vi "read position.vi"(8 "error in (no error)":errorcluster, 11 "Stepper in":refnum<class "Stepper.lvclass">) -> (0 "error out":errorcluster, 2 "Angle":dbl, 3 "Stepper out":refnum<class "Stepper.lvclass">)   [LabVIEW 2025, in "Motor.lvlib" / "Stepper.lvclass"]
uses:
  Stepper.lvclass
  Stepper.lvclass/Stepper.ctl
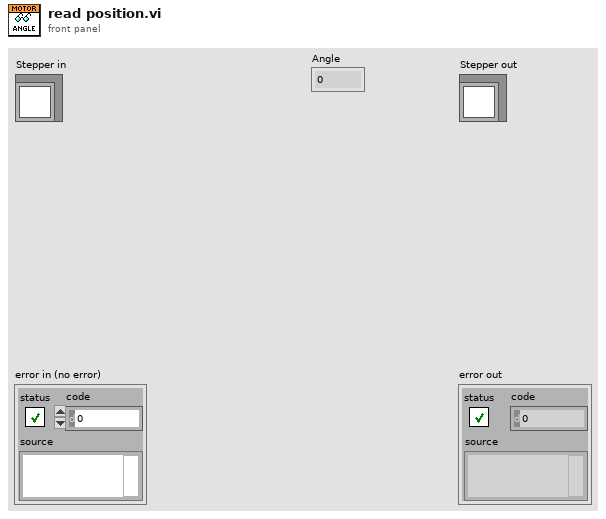
[diagram p1: front panel]
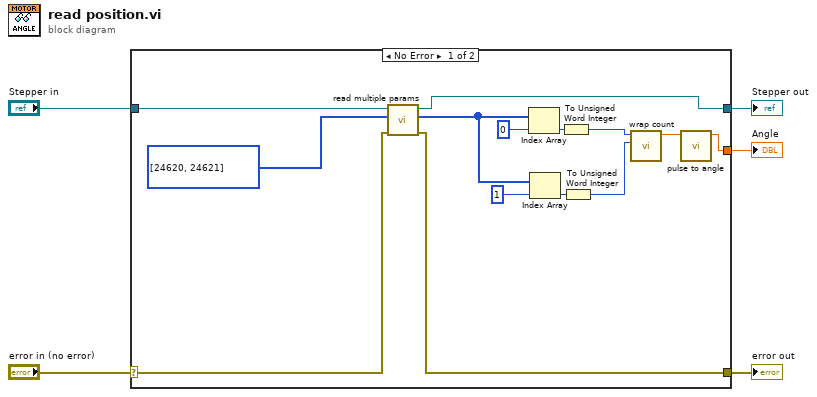
[diagram p0: block diagram]
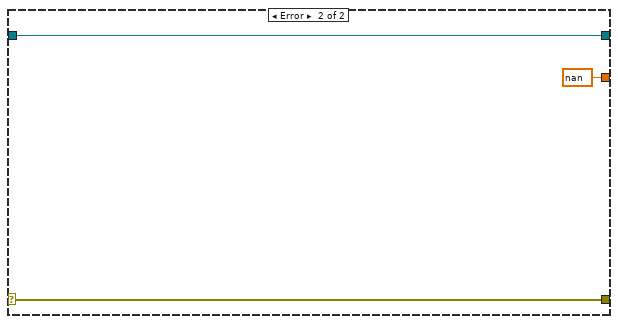
[diagram p2: hidden frame]
diagram:
  n1 = case shown="No Error" "error in (no error)" {
    selector: "error in (no error)" -> [w17 w22]
    tunnel: [w12 w22] -> w4
    tunnel: [w13 w21] -> w2
    tunnel: "Stepper in" -> [w19 w21]
    tunnel: [w11 nan ("Angle")] -> w1
    frame No Error {
      n2 = call-dynamic "read multiple params.vi"("error in (no error)"=w17, "Parameters"=u32[] [24620, 24621], "Stepper in"=w19) -> ("error out"=w12:errorcluster, "Hex Result"=w14:u32[], "Stepper out"=w13:refnum<class "Stepper.lvclass">)  [unwired: 6 in]
      n3 = Index Array(array=w14, index=0) -> (element=w9:u32)
      n4 = Index Array(array=w14, index=1) -> (element=w10:u32)
      n5 = To Unsigned Word Integer(number=w9) -> (unsigned 16bit integer=w7:u16)
      n6 = To Unsigned Word Integer(number=w10) -> (unsigned 16bit integer=w6:u16)
      n7 = call "wrap count.vi"("lo"=w6, "hi"=w7) -> ("Numeric"=w8:dbl)  [unwired: 9 in]
      n8 = call "pulse to angle.vi"("Pulses"=w8) -> ("Angle"=w11:dbl)  [unwired: 10 in]
    }
    frame Error {
    }
  }
  "error out" <- w4
  "Stepper out" <- w2
  "Angle" <- w1
